vi "OpenCOM.vi"(2 "error in (no error)":errorcluster, 3 "baud rate":u32=115200, 4 "VISA resource name":refnum<visa-resource-name>="COM7") -> (0 "error out":errorcluster, 1 "VISA resource name out":refnum<visa-resource-name>)   [LabVIEW 2012, in "NFC Driver.lvlib"]
uses:
  NFC Driver.lvlib
  <vilib>/Instr/_visa.llb/VISA Configure Serial Port (Instr).vi
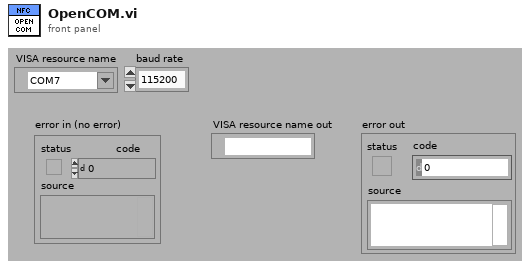
[diagram p1: front panel]
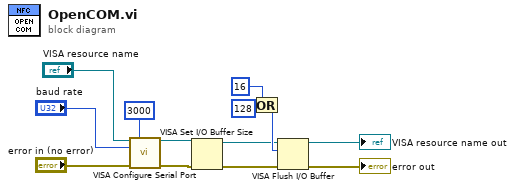
[diagram p0: block diagram]
diagram:
  n1 = call-poly "VISA Configure Serial Port"("VISA resource name"="VISA resource name", "timeout (10sec)"=u32 3000, "baud rate (9600)"="baud rate", "error in (no error)"="error in (no error)") -> ("VISA resource name out"=w8:refnum<visa-resource-name>, "error out"=w7:errorcluster)  [unwired: 10 in]
  n2 = VISA Set I/O Buffer Size(VISA resource name=w8, error in (no error)=w7) -> (VISA resource name out=w10:refnum<visa-resource-name>, error out=w9:errorcluster)  [unwired: 2 in]
  n3 = Or(x=u32 16 ("timeout (10sec)"), y=u32 128 ("timeout (10sec)")) -> (x .or. y?=w11:u32)
  n4 = VISA Flush I/O Buffer(VISA resource name=w10, mask (16)=w11, error in (no error)=w9) -> (VISA resource name out=→"VISA resource name out":refnum<visa-resource-name>, error out=→"error out":errorcluster)
